vi "Transport_Read_Plot.vi"(6 "Transport Graph Properties":T1={"Transport Line Size"=0, "Transport Line Color"=16774656} {"Transport Line Size" items=["Extra Small", "Small", "Medium", "Large", "Extra Large"]}, 7 "default (0 dbl)":ext format="%.2e", 9 "Transport File Path":path) -> (2 "Transport":cluster{ext[], ext[]}[](graph), 3 "Transport File":path)   [LabVIEW 2015]
uses:
  <vilib>/Utility/file.llb/Read Delimited Spreadsheet (string).vi
panel:
  out "Array 2":ext[][](array[numeric])
  out "Array":ext[][](array[numeric])
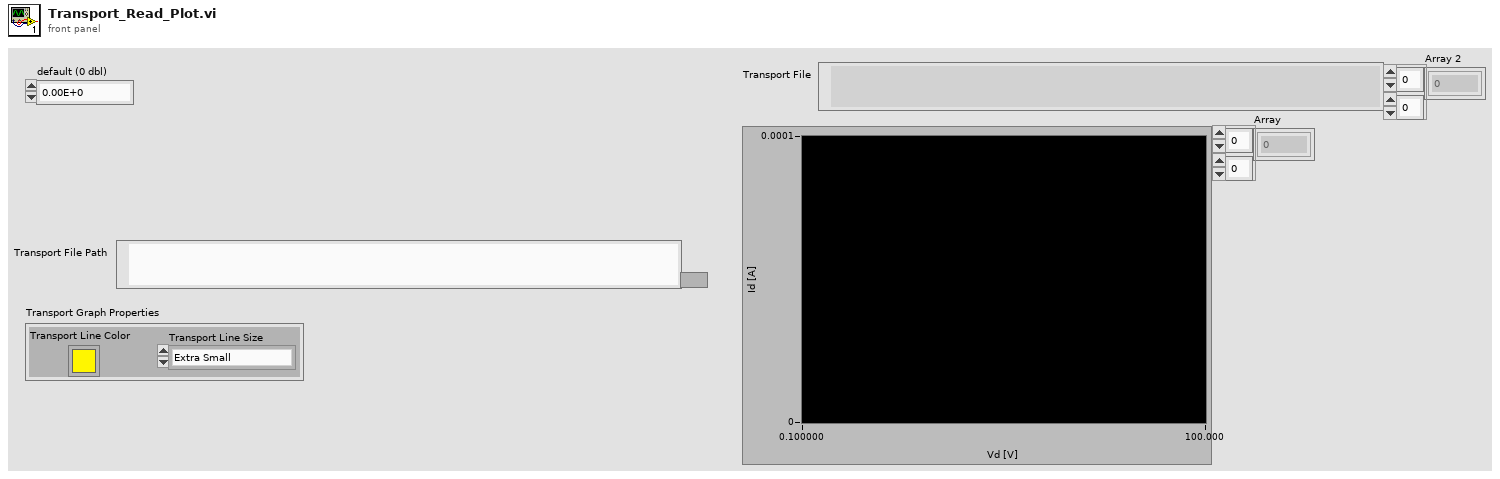
[diagram p1: front panel]
types:
  T1 = cluster{"Transport Line Size":u16, "Transport Line Color":u32}
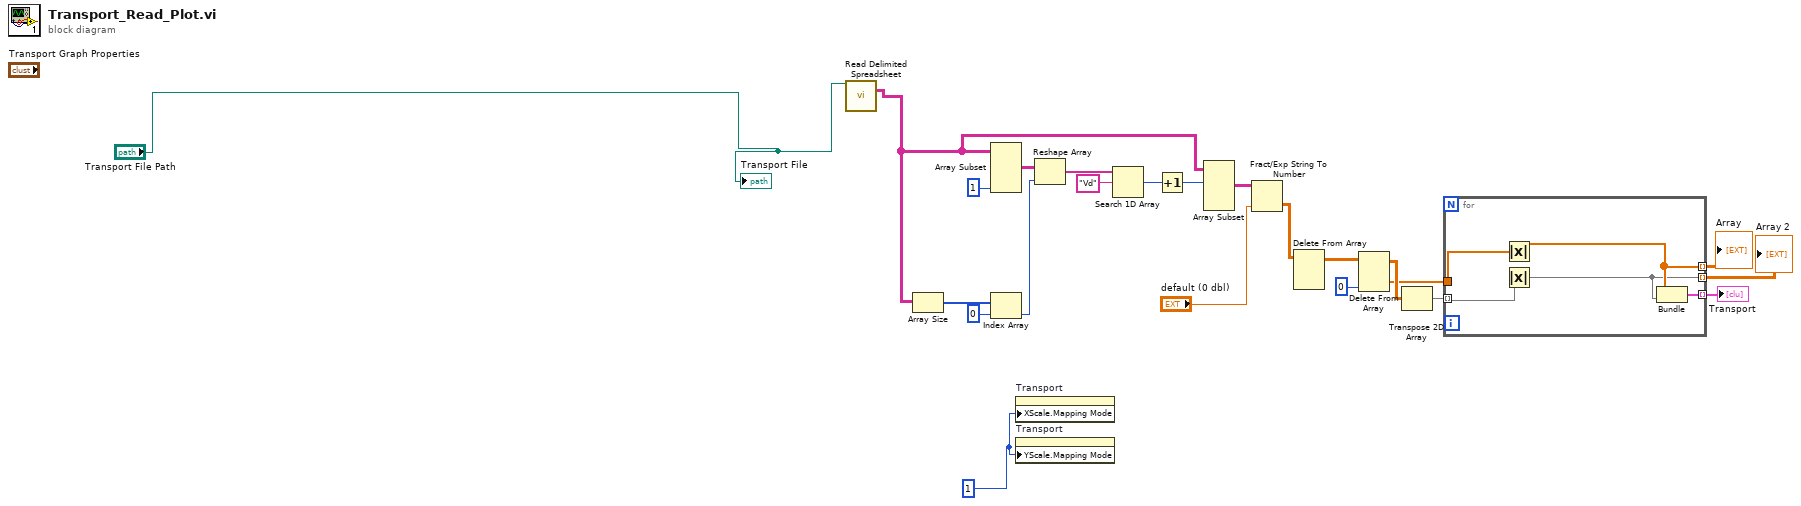
[diagram p0: block diagram]
diagram:
  w3 = 1
  n1 = call-poly <vilib>:"Read Delimited Spreadsheet.vi"("file path (dialog if empty)"="Transport File Path") -> ("all rows"=w5:string[][])  [unwired: 9 in, 5 out]
  n2 = Array Size(array=w5) -> (size(s)=w23:i32[])
  n3 = Array Subset(array=w5, length (col)=1) -> (w19:string[][])  [unwired: 3 in]
  n4 = Index Array(array=w23, index=0) -> (element=w13:i32)
  n5 = property on="Transport" class="XYGraph (strict)"("XScale.Mapping Mode"=w3) -> ()  [unwired: 2 in, 2 out]
  n6 = property on="Transport" class="XYGraph (strict)"("YScale.Mapping Mode"=w3) -> ()  [unwired: 2 in, 2 out]
  n7 = Reshape Array(w19, w13) -> (w18:string[])
  n8 = Search 1D Array(1D array=w18, element="Vd") -> (index of element=w17:i32)  [unwired: 1 in]
  n9 = Increment(x=w17) -> (x+1=w16:i32)
  n10 = Array Subset(array=w5, index (row)=w16) -> (w14:string[][])  [unwired: 3 in]
  n11 = Fract/Exp String To Number(string=w14, default (0 dbl)="default (0 dbl)") -> (number=w8:ext[][])  [unwired: 2 in, 1 out]
  n12 = Delete From Array(array=w8) -> (array with subset deleted=w7:ext[][])  [unwired: 3 in, 1 out]
  n13 = Delete From Array(array=w7, index (col)=0 ("Deaktivierter Index (Spalte)")) -> (deleted portion=w10:ext[], array with subset deleted=w11:ext[][])  [unwired: 2 in]
  n14 = Transpose 2D Array(2D array=w11) -> (transposed array=w12:ext[][])
  n15 = for {
    tunnel: w10 -> [w27]
    tunnel: w12 -> [w26] mode=indexing
    tunnel: [w28] -> w6 mode=indexing
    tunnel: [w25] -> w2 mode=indexing
    tunnel: [w24] -> w1 mode=indexing
    n16 = Absolute Value(x=w27) -> (abs(x)=w25:ext[])
    n17 = Absolute Value(x=w26) -> (abs(x)=w24:ext[])
    n18 = Bundle(w25, w24) -> (w28:cluster{ext[], ext[]})  [unwired: 1 in]
  }
  "Transport" <- w6
  "Array" <- w2
  "Array 2" <- w1
  "Transport File" <- "Transport File Path"
